vi "Roughing Valve Precheck Selection.vi"(10 "Isolate HPBD":bool, 11 "Chamber Selection":T1) -> (3 "States Out":string)   [LabVIEW 2011]
uses:
  Chamber Selection_typdef.ctl
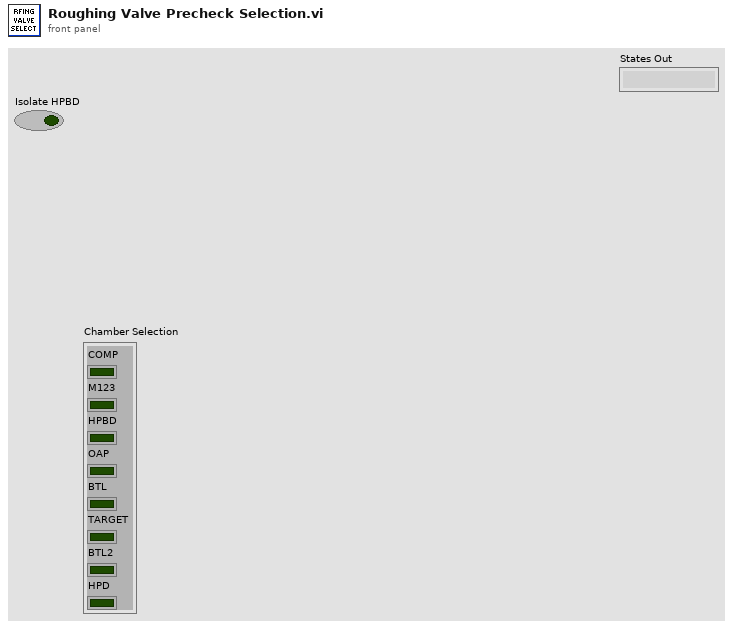
[diagram p1: front panel]
types:
  T1 = typedef "Chamber Selection_typdef.ctl" = cluster{"COMP":bool, "M123":bool, "HPBD":bool, "OAP":bool, "BTL":bool, "TARGET":bool, "BTL2":bool, "HPD":bool}
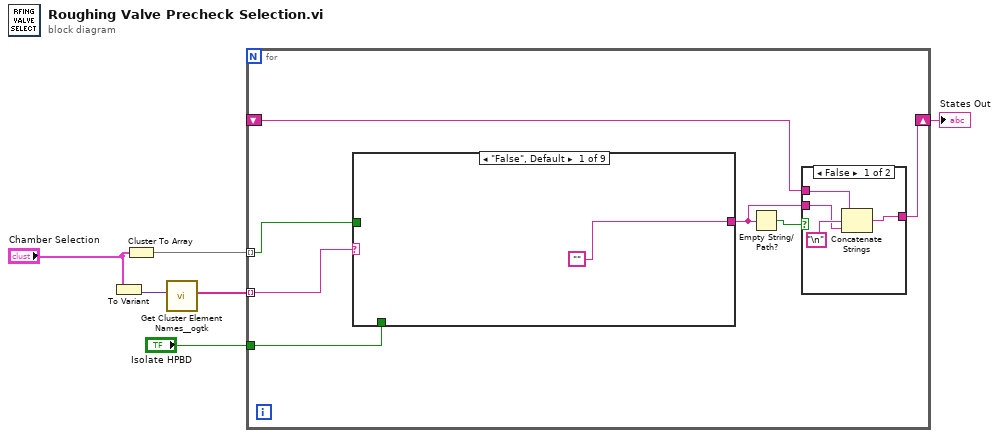
[diagram p0: block diagram]
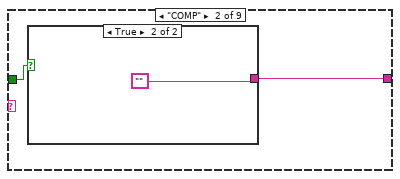
[diagram p3: hidden frame]
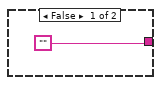
[diagram p4: hidden frame]
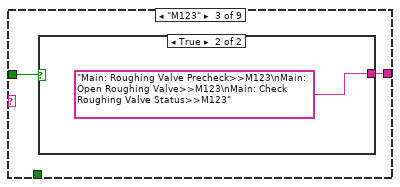
[diagram p5: hidden frame]
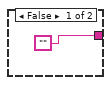
[diagram p6: hidden frame]
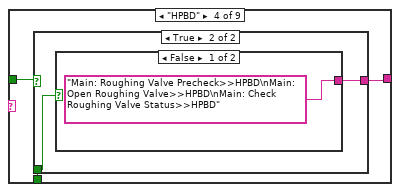
[diagram p7: hidden frame]
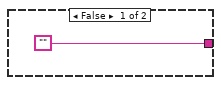
[diagram p8: hidden frame]
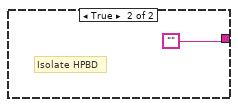
[diagram p9: hidden frame]
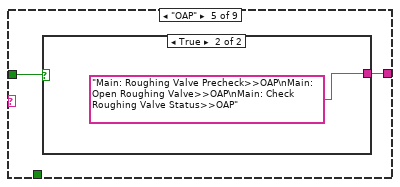
[diagram p10: hidden frame]
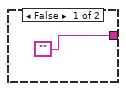
[diagram p11: hidden frame]
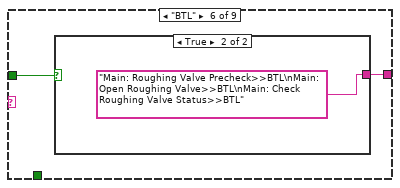
[diagram p12: hidden frame]
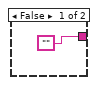
[diagram p13: hidden frame]
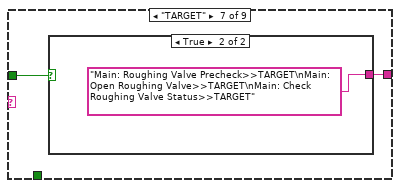
[diagram p14: hidden frame]
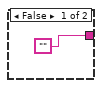
[diagram p15: hidden frame]
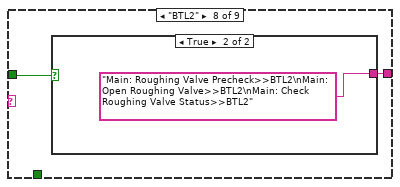
[diagram p16: hidden frame]
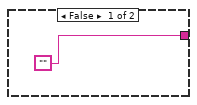
[diagram p17: hidden frame]
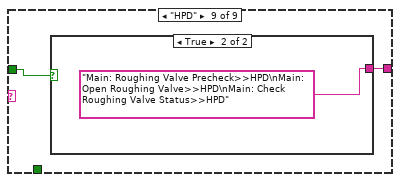
[diagram p18: hidden frame]
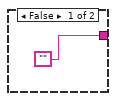
[diagram p19: hidden frame]
diagram:
  n1 = To Variant(anything="Chamber Selection") -> (Variant=w4:variant)
  n2 = Cluster To Array(cluster="Chamber Selection") -> (array=w3:bool[])
  n3 = call <userlib>:"Get Cluster Element Names__ogtk.vi"("Cluster"=w4) -> ("Element Names"=w5:string[])  [unwired: 9 in, 1 out]
  n4 = for {
    tunnel: w3 -> [w12] mode=indexing
    tunnel: w5 -> [w13] mode=indexing
    tunnel: "Isolate HPBD" -> [w7]
    shift-right: [w9] -> w1
    shift-left: _ -> [w8]
    n5 = case shown="\"False\", Default" w13 {
      tunnel: w12 -> [_ w21 w24 w30 w37 w40 w45 w48 w52]
      tunnel: ["" w20 w25 w28 w36 w41 w44 w49 w53] -> w10
      tunnel: w7 -> [_ _ _ w29 _ _ _ _ _]
      frame "False", Default {
      }
      frame "COMP" {
        n6 = case shown="True" w21 {
          tunnel: ["" ""] -> w20
          frame False {
          }
          frame True {
          }
        }
      }
      frame "M123" {
        n7 = case shown="True" w24 {
          tunnel: ["" "Main: Roughing Valve Precheck>>M123\nMain: Open Roughing Valve>>M123\nMain: Check Roughing Valve Status>>M123"] -> w25
          frame False {
          }
          frame True {
          }
        }
      }
      frame "HPBD" {
        n8 = case shown="True" w30 {
          tunnel: ["" w32] -> w28
          tunnel: w29 -> [_ w33]
          frame False {
          }
          frame True {
            n9 = case shown="False" w33 {
              tunnel: ["Main: Roughing Valve Precheck>>HPBD\nMain: Open Roughing Valve>>HPBD\nMain: Check Roughing Valve Status>>HPBD" ""] -> w32
              frame False {
              }
              frame True {
                # "Isolate HPBD"
              }
            }
          }
        }
      }
      frame "OAP" {
        n10 = case shown="True" w37 {
          tunnel: ["" "Main: Roughing Valve Precheck>>OAP\nMain: Open Roughing Valve>>OAP\nMain: Check Roughing Valve Status>>OAP"] -> w36
          frame False {
          }
          frame True {
          }
        }
      }
      frame "BTL" {
        n11 = case shown="True" w40 {
          tunnel: ["" "Main: Roughing Valve Precheck>>BTL\nMain: Open Roughing Valve>>BTL\nMain: Check Roughing Valve Status>>BTL"] -> w41
          frame False {
          }
          frame True {
          }
        }
      }
      frame "TARGET" {
        n12 = case shown="True" w45 {
          tunnel: ["" "Main: Roughing Valve Precheck>>TARGET\nMain: Open Roughing Valve>>TARGET\nMain: Check Roughing Valve Status>>TARGET"] -> w44
          frame False {
          }
          frame True {
          }
        }
      }
      frame "BTL2" {
        n13 = case shown="True" w48 {
          tunnel: ["" "Main: Roughing Valve Precheck>>BTL2\nMain: Open Roughing Valve>>BTL2\nMain: Check Roughing Valve Status>>BTL2"] -> w49
          frame False {
          }
          frame True {
          }
        }
      }
      frame "HPD" {
        n14 = case shown="True" w52 {
          tunnel: ["" "Main: Roughing Valve Precheck>>HPD\nMain: Open Roughing Valve>>HPD\nMain: Check Roughing Valve Status>>HPD"] -> w53
          frame False {
          }
          frame True {
          }
        }
      }
    }
    n15 = Empty String/Path?(string/path=w10) -> (empty?=w11:bool)
    n16 = case shown="False" w11 {
      tunnel: w10 -> [w14 w18]
      tunnel: [w16 w18] -> w9
      tunnel: w8 -> [w15 _]
      frame False {
        n17 = Concatenate Strings(w15, "\n", w14) -> (w16:string)
      }
      frame True {
      }
    }
  }
  "States Out" <- w1
